vi "UserSettings.vi"() -> ()   [LabVIEW 2011]
uses:
  Strict Type Controls/Settings.ctl
  Strict Type Controls/Settings Operation.ctl
panel:
  in  "Cancel":bool
  in  "OK":bool
  in  "Settings":T1={"DMM Settings"={"Port"="", "baud rate"=9600, "data bits"=8, "stop bits"=10, "parity"=enum."None", "flow control"=enum."None"}, "Modbus Settings"={"Port"="", "baud rate"=9600, "parity"=enum."None", "flow control"=enum."None"}} {"DMM Settings"."data bits" min=5 max=8 step=1}
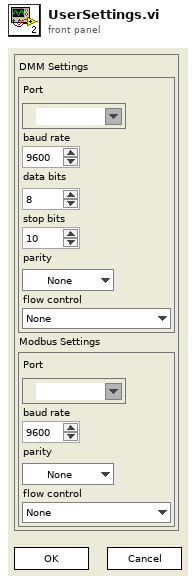
[diagram p1: front panel]
types:
  T1 = typedef "Settings.ctl" = cluster{"DMM Settings":cluster{"Port":refnum<visa-resource-name>, "baud rate":u32, "data bits":u16, "stop bits":u16, "parity":enum16{"None", "Odd", "Even", "Mark", "Space"}, "flow control":enum16{"None", "XON/XOFF", "RTS/CTS", "XON/XOFF & RTS/CTS", "DTR/DSR", "XON/XOFF & DTR/DSR"}}, "Modbus Settings":cluster{"Port":refnum<visa-resource-name>, "baud rate":u32, "parity":enum16{"None", "Odd", "Even", "Mark", "Space"}, "flow control":enum16{"None", "XON/XOFF", "RTS/CTS", "XON/XOFF & RTS/CTS", "DTR/DSR", "XON/XOFF & DTR/DSR"}}}
  T2 = enum32{"invalid app kind", "Development System", "Run Time System", "Student Edition", "Embedded LabVIEW", "Evaluation", "Custom"}
  T3 = typedef "Settings Operation.ctl" = enum8{"Get Value", "Set Value", "Read File", "Write File", "Write Stored Value"}
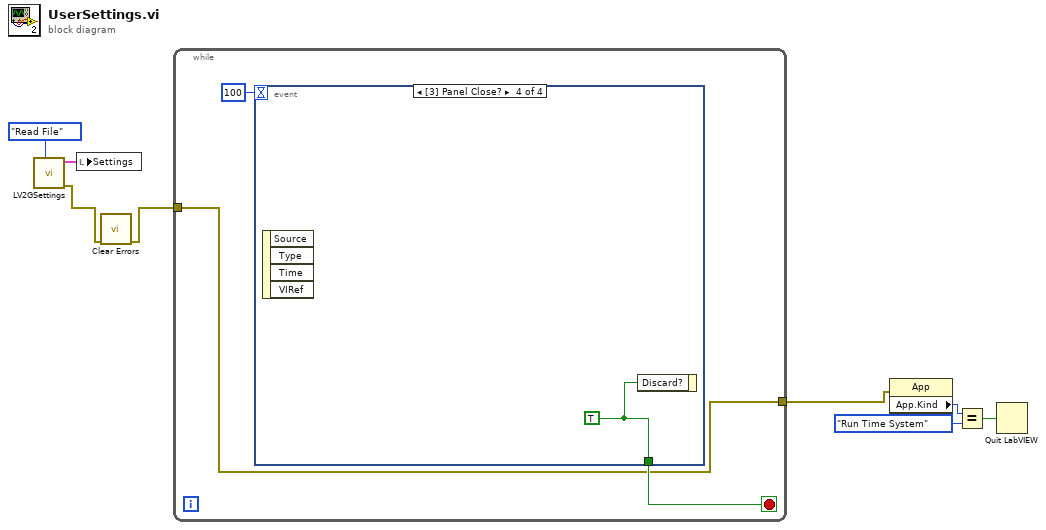
[diagram p0: block diagram]
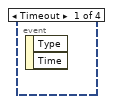
[diagram p2: hidden frame]
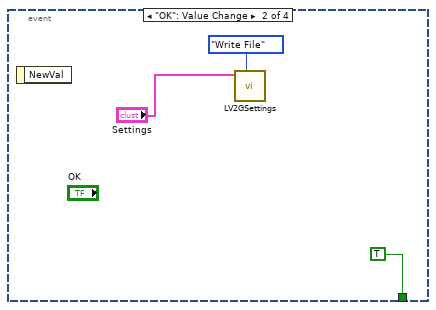
[diagram p3: hidden frame]
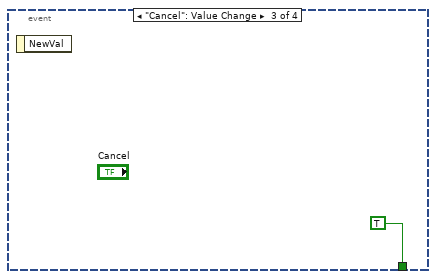
[diagram p4: hidden frame]
diagram:
  n1 = call "LV2GSettings.vi"("Operation"=Settings_Operation."Read File") -> ("error out"=w2:errorcluster, "Settings out"=w7:T1)  [unwired: 2 in, 7 out]
  n2 = local write "Settings"(w7) -> ()
  n3 = call <vilib>:"Clear Errors.vi"("error in (no error)"=w2) -> ("error out"=w1:errorcluster)  [unwired: 6 out]
  n4 = while {
    tunnel: w1 -> [w9]
    tunnel: [w9] -> w3
    stop <- w10 stop-if-true
    n5 = event shown="[3] Panel Close?" {
      selector: _ -> [_ _ _ _]
      dyn-events: _ -> [_ _ _ _]
      timeout: 100 -> [_ _ _ _]
      tunnel: [_ TRUE TRUE w16] -> w10
      event Timeout {
        n6 = event-data() -> ()  [unwired: 3 out]
      }
      event "OK": Value Change {
        n7 = event-data() -> ()  [unwired: 2 out]
        n8 = call "LV2GSettings.vi"("Operation"=Settings_Operation."Write File", "Settings"="Settings") -> ()  [unwired: 1 in, 9 out]
      }
      event "Cancel": Value Change {
        n9 = event-data() -> ()  [unwired: 2 out]
      }
      event Panel Close? {
        w16 = TRUE
        n10 = event-data() -> ()  [unwired: 5 out]
        n11 = event-data("Discard?"=w16) -> ()  [unwired: 1 in, 1 out]
      }
    }
  }
  n12 = property class="App"(error in=w3) -> ("App.Kind"=w6:T2)  [unwired: 1 in, 2 out]
  n13 = Equal?(x=w6, y=T2."Run Time System" ("Application:Kind")) -> (x = y?=w4:bool)
  n14 = Quit LabVIEW(quit? (T)=w4) -> ()
